vi "Write Axi.In.vi"(8 "error in (no error)":errorcluster, 10 "Axi.In":T1, 11 "Ethernet MAC - Custom in":refnum<class "Ethernet MAC - Custom.lvclass">) -> (0 "error out":errorcluster, 3 "Ethernet MAC - Custom out":refnum<class "Ethernet MAC - Custom.lvclass">)   [LabVIEW 2020, in "Ethernet MAC - Custom.lvclass"]
uses:
  Ethernet MAC - Custom.lvclass
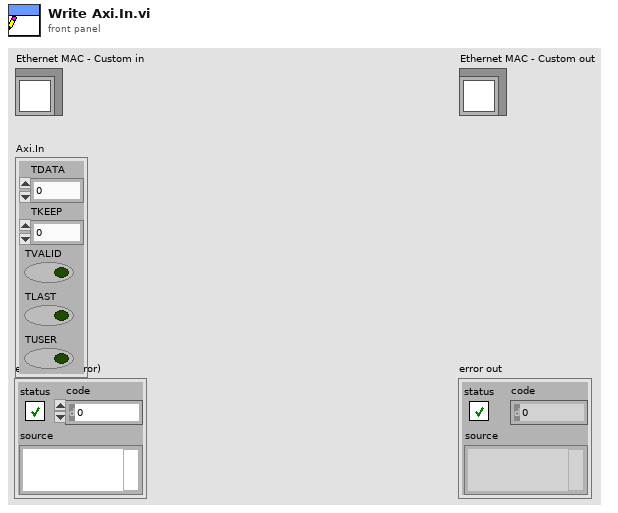
[diagram p1: front panel]
types:
  T1 = cluster{"TDATA":u64, "TKEEP":u8, "TVALID":bool, "TLAST":bool, "TUSER":bool}
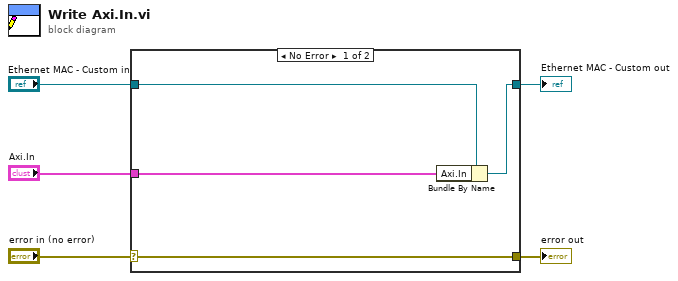
[diagram p0: block diagram]
diagram:
  n1 = case shown="No Error" "error in (no error)" {
    selector: "error in (no error)" -> [w9 w10]
    tunnel: [w9 w10] -> w4
    tunnel: [w7 w11] -> w2
    tunnel: "Ethernet MAC - Custom in" -> [w8 w11]
    tunnel: "Axi.In" -> [w6 _]
    frame No Error {
      n2 = Bundle By Name(cluster=w8, "Axi.In"=w6) -> (w7:refnum<class "Ethernet MAC - Custom.lvclass">)
    }
    frame Error {
    }
  }
  "error out" <- w4
  "Ethernet MAC - Custom out" <- w2
